vi "Python_Interface.vi"() -> ()   [LabVIEW 2024]
panel:
  out "Boolean":bool
  in  "Boolean 2":bool
  in  "Python version":string
  in  "function name":string
  in  "module path":path
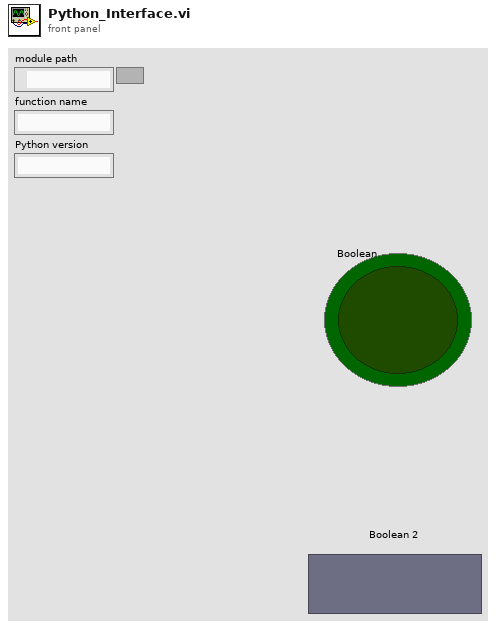
[diagram p1: front panel]
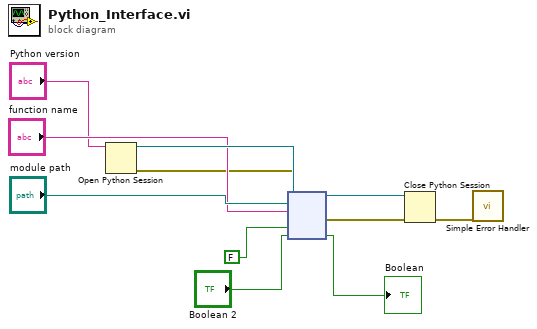
[diagram p0: block diagram]
diagram:
  n1 = Open Python Session(python version="Python version") -> (session out=w11:refnum<k35>, error out=w3:errorcluster)  [unwired: 2 in]
  n2 = node(w11, "module path", "function name", w3, FALSE, "Boolean 2") -> (w10:refnum<k35>, w9:errorcluster, →"Boolean":bool)  [unwired: 1 in, 2 out]
  n3 = Close Python Session(session in=w10, error in=w9) -> (11:w5:errorcluster)
  n4 = call <vilib>:"Simple Error Handler.vi"("error in (no error)"=w5) -> ()  [unwired: 4 in, 5 out]
